vi "Configure RF Markers.vi"(0 "VISA resource name":refnum<visa-resource-name>, 1 "Peak Threshold (-50.0 dBm)":dbl=-50.0, 2 "Peak Excursion (30.0 dBm)":dbl=30.0, 5 "Enable Manual Markers (F: Disabled)":bool, 7 "Enable Peak Markers (T: Enabled)":bool=TRUE, 9 "Maximum Peak Markers (5)":i32=5, 11 "error in (no error)":errorcluster, 12 "Manual Marker A Frequency (0 Hz)":dbl, 13 "Manual Marker B Frequency (0 Hz)":dbl) -> (4 "VISA resource name out":refnum<visa-resource-name>, 15 "error out":errorcluster)   [LabVIEW 2016, in "Tektronix DPO MSO 2000 4000 Series.lvlib"]
doc: "Configures the RF markers to automatically or manually locate peaks and sets the maximum number of peaks to mark.\n\n<B>Note:</B>\nOnly valid in <B>MDO</B> series instruments"
uses:
  Tektronix DPO MSO 2000 4000 Series.lvlib
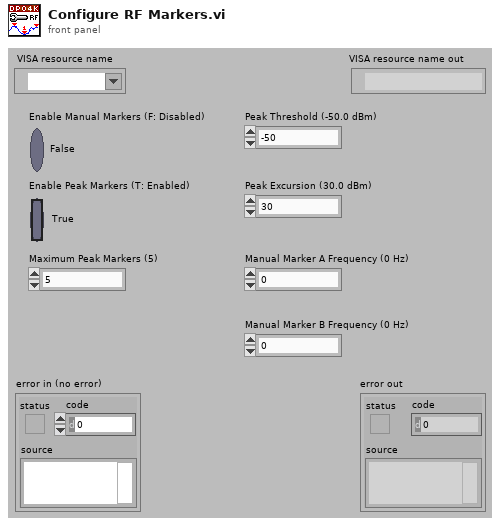
[diagram p1: front panel]
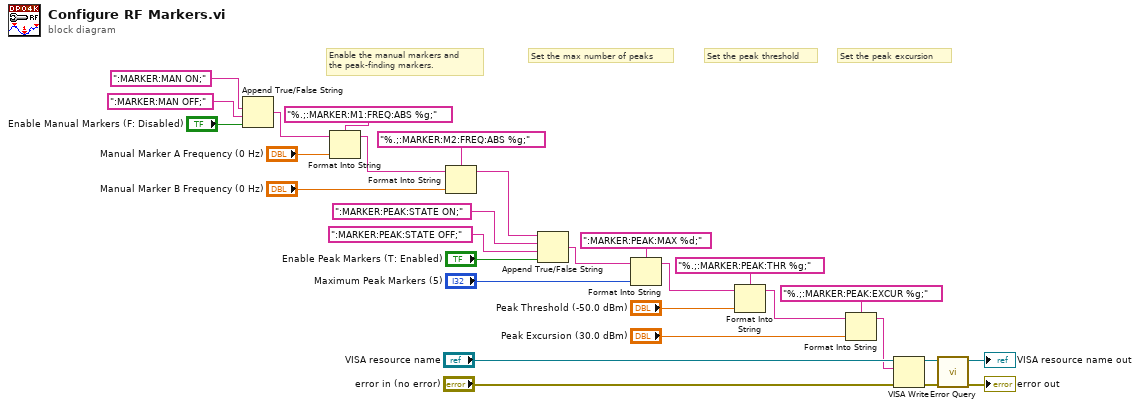
[diagram p0: block diagram]
diagram:
  # "Set the peak excursion"
  # "Set the peak threshold"
  # "Set the max number of peaks"
  # "Enable the manual markers and \nthe peak-finding markers."
  n1 = Append True/False String(1:"Enable Manual Markers (F: Disabled)", 2:":MARKER:MAN OFF;" ("false string"), 3:":MARKER:MAN ON;" ("false string")) -> (0:w1:string)  [unwired: 1 in]
  n2 = Format Into String(format string="%.;:MARKER:M1:FREQ:ABS %g;", initial string=w1, "Manual Marker A Frequency (0 Hz)") -> (resulting string=w4:string)  [unwired: 1 in, 1 out]
  n3 = Format Into String(format string="%.;:MARKER:M2:FREQ:ABS %g;", initial string=w4, "Manual Marker B Frequency (0 Hz)") -> (resulting string=w2:string)  [unwired: 1 in, 1 out]
  n4 = Append True/False String(1:"Enable Peak Markers (T: Enabled)", 2:":MARKER:PEAK:STATE OFF;" ("false string"), 3:":MARKER:PEAK:STATE ON;" ("true string"), 4:w2) -> (0:w14:string)
  n5 = Format Into String(format string=":MARKER:PEAK:MAX %d;", initial string=w14, "Maximum Peak Markers (5)") -> (resulting string=w17:string)  [unwired: 1 in, 1 out]
  n6 = Format Into String(format string="%.;:MARKER:PEAK:THR %g;", initial string=w17, "Peak Threshold (-50.0 dBm)") -> (resulting string=w21:string)  [unwired: 1 in, 1 out]
  n7 = Format Into String(format string="%.;:MARKER:PEAK:EXCUR %g;", initial string=w21, "Peak Excursion (30.0 dBm)") -> (resulting string=w22:string)  [unwired: 1 in, 1 out]
  n8 = VISA Write(VISA resource name="VISA resource name", write buffer=w22, error in (no error)="error in (no error)") -> (VISA resource name out=w26:refnum<visa-resource-name>, error out=w27:errorcluster)  [unwired: 1 out]
  n9 = call "Error Query.vi"("error in (no error)"=w27, "VISA resource name"=w26) -> ("error out"=→"error out":errorcluster, "VISA resource name out"=→"VISA resource name out":refnum<visa-resource-name>)  [unwired: 6 in, 2 out]
